vi "Average Waveform .vi"(10 "index":i32, 11 "Waveform Array":waveform(dbl)[](array[waveform])) -> (1 "VRECT Ripple":dbl, 2 "VRECT":dbl format="%0.2f")   [LabVIEW 2010]
uses:
  <vilib>/Analysis/NI_AALBase.lvlib
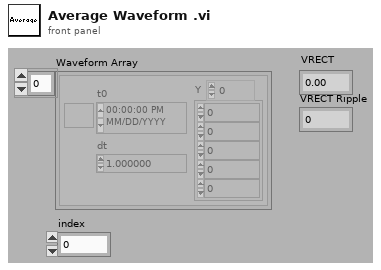
[diagram p1: front panel]
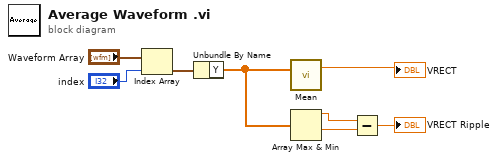
[diagram p0: block diagram]
diagram:
  n1 = Index Array(array="Waveform Array", index="index") -> (element=w3:waveform(dbl))
  n2 = Unbundle By Name(w3) -> ("Y"=w2:dbl[])
  n3 = call <vilib>:"Mean.vi"("X"=w2) -> ("mean"=→"VRECT":dbl)  [unwired: 1 out]
  n4 = Array Max & Min(array=w2) -> (max value=w8:dbl, min value=w7:dbl)  [unwired: 2 out]
  n5 = Subtract(x=w8, y=w7) -> (x-y=→"VRECT Ripple":dbl)
